vi "Get RootNodebyVIRef.vi"(8 "error in":errorcluster caption="错误输入（无错误）", 11 "vi*":refnum<vi>) -> (0 "error out":errorcluster, 3 "RootNode*":refnum<data-value>)   [LabVIEW 2016, in "PCM PanelSplit.lvclass"]
uses:
  PCM PanelSplit.lvclass
  PanelSplitToolkit/PanelRootNode/PanelRootNode.lvclass
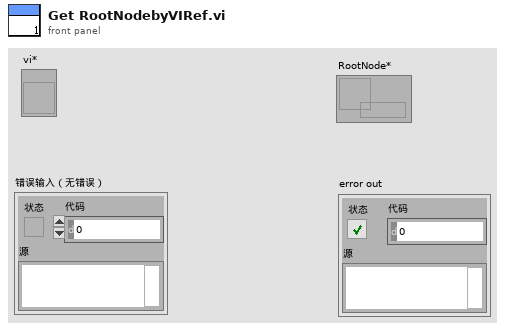
[diagram p1: front panel]
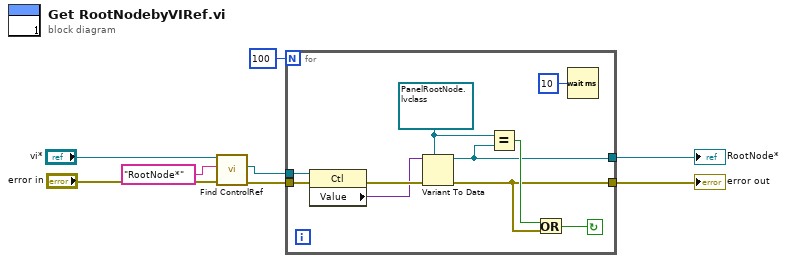
[diagram p0: block diagram]
diagram:
  n1 = call "Find ControlRef.vi"("error in (no error)"="error in", "control name"="RootNode*", "vi*"="vi*") -> ("error out"=w5:errorcluster, "ctrl*"=w4:refnum<vi>)  [unwired: 6 in, 1 out]
  n2 = for {
    N: 100 -> [_]
    tunnel: w5 -> [w17]
    tunnel: w4 -> [w16]
    tunnel: [w11] -> w1
    tunnel: [w9] -> w2
    stop <- w10 continue-if-true
    w13 = refnum<data-value> refnum ("数据值引用")
    n3 = property class="Ctl"(reference=w16, error in=w17) -> (error out=w18:errorcluster, "Value"=w15:variant)  [unwired: 1 out]
    n4 = Variant To Data(error in=w18, type=w13, Variant=w15) -> (data=w9:refnum<data-value>, error out=w11:errorcluster)
    n5 = Equal?(x=w13, y=w9) -> (x = y?=w12:bool)
    n6 = Or(x=w12, y=w11) -> (x .or. y?=w10:bool)
    n7 = Wait (ms)(milliseconds to wait=u32 10 ("等待时间（毫秒）")) -> ()  [unwired: 1 out]
  }
  "RootNode*" <- w2
  "error out" <- w1
